vi "PV ActiveLine - Measurement Data - 2 Gauges.vi"(8 "Fehler (Eingang)":errorcluster, 11 "Referenz in":refnum<visa-resource-name>) -> (0 "Cluster (Ausgang)":errorcluster, 1 "Pressure Sensor 2":dbl format="%.3e", 2 "Pressure Sensor 1":dbl format="%.3e", 3 "Referenz out":refnum<visa-resource-name>, 4 "Status Sensor 2":i32(ring) items=["data OK", "underrange", "overrange", "sensor error", "sensor off", "no sensor", "ID error"], 5 "Status Sensor 1":i32(ring) items=["data OK", "underrange", "overrange", "sensor error", "sensor off", "no sensor", "ID error"])   [LabVIEW 2013, in "PV ActiveLine.lvlib"]
doc: "PRX - Measurement Data Gauges 1 and 2\n\nReceive: a,sx.xxxxEsxx,b,sy.yyyyEsyy\n\nStatus gauge 1,\na =\n0 –> Measurement data okay\n1 –> Underrange\n2 –> Overrange\n3 –> Sensor error\n4 –> Sensor off (IKR, PKR, IMR, PBR)\n5 –> No sensor (output: 5,2.0000E-2 [hPa])\n6 –> Identification error\nMeasurement value gauge 1 [in current pressure unit]\nStatus gauge 2,\nb= \nMeasurement value gauge 2 [in current pressure unit]\n\nValues always in exponential format.\nFor logarithmic gauges, the 3rd and 4th decimal are always 0."
uses:
  PV ActiveLine.lvlib
panel:
  # "mbar"
  # "mbar"
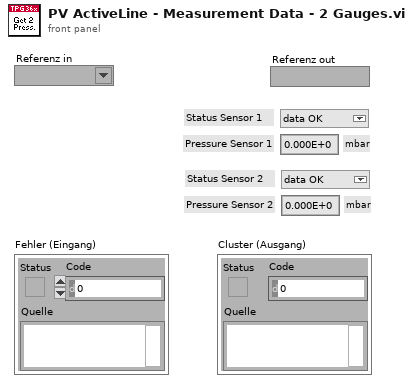
[diagram p1: front panel]
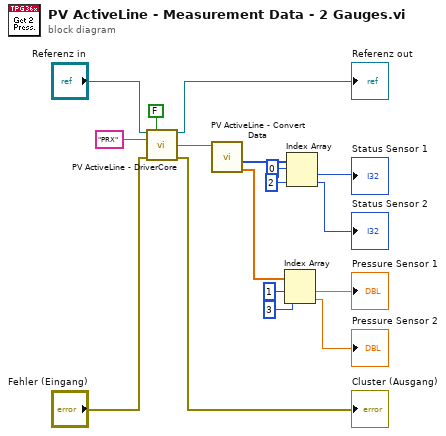
[diagram p0: block diagram]
diagram:
  n1 = call "PV ActiveLine - DriverCore.vi"("Referenz in"="Referenz in", "Write/Read"=FALSE, "Command"="PRX", "Fehler (Eingang)"="Fehler (Eingang)") -> ("Referenz out"=→"Referenz out":refnum<visa-resource-name>, "String Out"=w11:string, "Cluster (Ausgang)"=→"Cluster (Ausgang)":errorcluster)  [unwired: 9 in]
  n2 = call "PV ActiveLine - Convert Data.vi"("String in"=w11) -> ("DBL out"=w10:dbl[], "Integer Out"=w9:i32[])  [unwired: 7 in, 2 out]
  n3 = Index Array(array=w10, index #1=1 ("Index"), index #2=3 ("Index")) -> (element #1=→"Pressure Sensor 1":dbl, element #2=→"Pressure Sensor 2":dbl)
  n4 = Index Array(array=w9, index #1=0 ("Index"), index #2=2 ("Index")) -> (element #1=→"Status Sensor 1":i32, element #2=→"Status Sensor 2":i32)
